vi "LogFile schreiben pruefen.vi"(11 "LogDatei erstellen":bool) -> (0 "LogFile schreiben?":bool, 3 "LogDatei erstellen":bool)   [LabVIEW 2020, in "LogKonfig.lvlib"]
uses:
  LogKonfig.lvlib
  Aktionen Logdatei erstellen.ctl
  Aktionen Trigger.ctl
  cRIO/PC/Kommunikation mit cRIO.lvlib
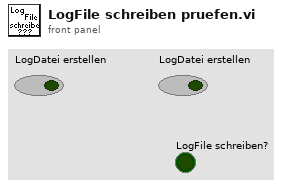
[diagram p1: front panel]
types:
  T1 = typedef "LogKonfig.lvlib/Aktionen Trigger.ctl" = enum16{"lesen", "ALLE schreiben", "Trigger prüfen", "Trigger rücksetzen"}
  T2 = typedef "LogKonfig.lvlib/Aktionen Logdatei erstellen.ctl" = enum16{"lesen", "Logdatei erstellen NEU", "Name NEU", "Pfad NEU", "Log Stop", "max Size"}
  T3 = typedef "LogKonfig.lvlib/Auswahlfeld aktiviert-deaktiviert.ctl" = u16
  T4 = typedef "Verwaltung - cRIO.lvlib/Digital Eingaenge 0-15.ctl" = cluster{"I0: N2 Nachf. FT-IR voll":bool, "I1: N2 Nachf. Vorrat leer":bool, "I2: (Klimaanlage eingeschaltet)":bool, "I3: (Klimaanlage Störung)":bool, "I4: Trigger Eingang (Messdaten sp.)":bool, "I5: Reserve":bool, "I6: Reserve":bool, "I7: Reserve":bool, "I8: Druckschalter Versorgung ok":bool, "I9: Reserve":bool, "I10: Reserve":bool, "I11: Reserve":bool, "I12: Drucksch. N2 Versorgung":bool, "I13: Reserve":bool, "I14: Drucksch. N2 Optikbox":bool, "I15: (Füllstand Kondensatbehälter)":bool}
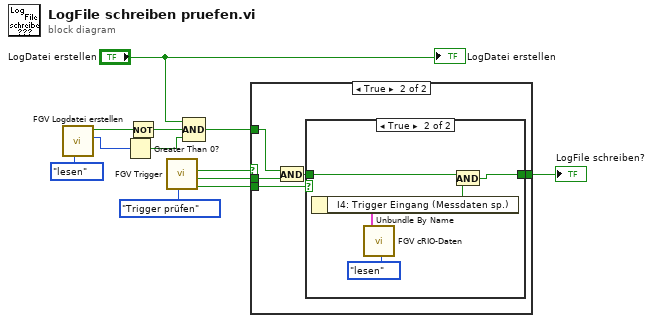
[diagram p0: block diagram]
diagram:
  n1 = call "FGV Logdatei erstellen.vi"("Aktion"=Aktionen_Logdatei_erstellen."lesen") -> ("Logdatei erstellen neu"=w3:T3, "Loggen stoppen"=w11:bool)  [unwired: 6 in, 3 out]
  n2 = Greater Than 0?(x=w3) -> (x > 0?=w2:bool)
  n3 = Not(x=w11) -> (.not. x?=w10:bool)
  n4 = call "FGV Trigger.vi"("Aktion"=Aktionen_Trigger."Trigger prüfen") -> ("Trigger Eingang"=w5:bool, "Trigger gesetzt?"=w6:bool, "Trigger verwenden"=w8:bool)  [unwired: 7 in, 1 out]
  n5 = Compound Arithmetic op=AND("LogDatei erstellen", w10, w2) -> (w7:bool)
  n6 = case shown="True" w8 {
    tunnel: w7 -> [w13 w17]
    tunnel: w6 -> [_ w18]
    tunnel: w5 -> [_ w16]
    tunnel: [w13 w14] -> w4
    frame False {
    }
    frame True {
      n7 = And(x=w17, y=w18) -> (x .and. y?=w15:bool)
      n8 = case shown="True" w16 {
        tunnel: w15 -> [w19 w24]
        tunnel: [w19 w23] -> w14
        frame False {
        }
        frame True {
          n9 = call "FGV cRIO-Daten.vi"("Aktion"=enum16{"lesen", "schreiben"}."lesen") -> ("DI"=w21:T4)  [unwired: 9 in, 9 out]
          n10 = Unbundle By Name(w21) -> ("I4: Trigger Eingang (Messdaten sp.)"=w20:bool)
          n11 = And(x=w24, y=w20) -> (x .and. y?=w23:bool)
        }
      }
    }
  }
  "LogFile schreiben?" <- w4
  "LogDatei erstellen" <- "LogDatei erstellen"
